vi "_API_BINANCE_GET_BookTicker.vi"(0 "BinanceAPI in":refnum<class "BinanceAPI_.lvclass">, 5 "bookTicker":cluster{"symbol (eg. BTCUSDT)":string}={"symbol (eg. BTCUSDT)"="CAKEUSDT"}, 11 "error in (no error)":errorcluster) -> (4 "BinanceAPI out":refnum<class "BinanceAPI_.lvclass">, 6 "bookTicker":T1, 14 "Body":string, 15 "error out":errorcluster)   [LabVIEW 2022 SP3, in "BinanceAPI_.lvclass"]
doc: "https://binance-docs.github.io/apidocs/spot/en/#symbol-order-book-ticker"
uses:
  BinanceAPI_.lvclass
  BinanceAPI_.lvclass/BinanceAPI_.ctl
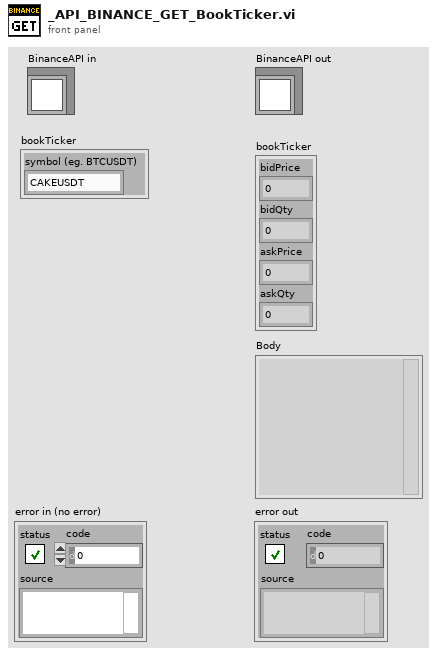
[diagram p1: front panel]
types:
  T1 = cluster{"bidPrice":dbl, "bidQty":dbl, "askPrice":dbl, "askQty":dbl}
  T2 = cluster{"bidPrice":string, "bidQty":string, "askPrice":string, "askQty":string}
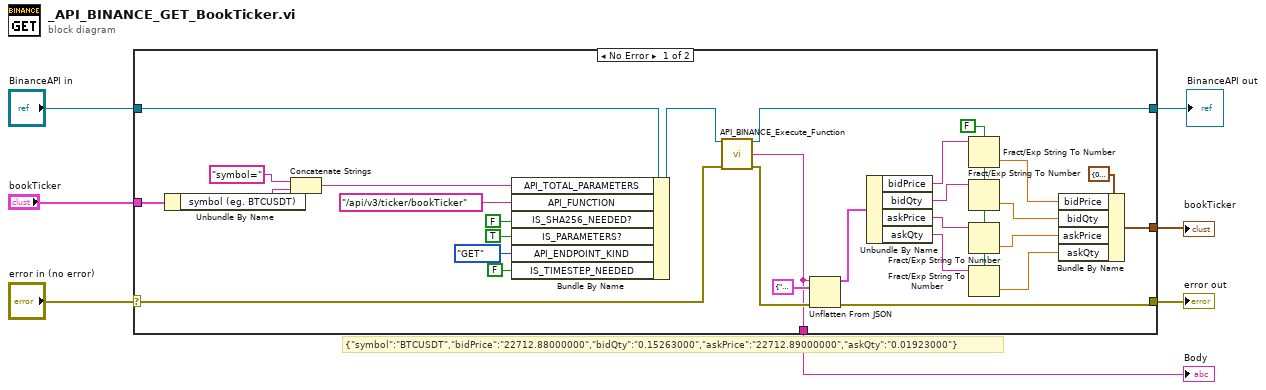
[diagram p0: block diagram]
diagram:
  # "{\"symbol\":\"BTCUSDT\",\"bidPrice\":\"22712.88000000\",\"bidQty\":\"0.15263000\",\"askPrice\":\"22712.89000000\",\"askQty\":\"0.01923000\"}"
  n1 = case shown="No Error" "error in (no error)" {
    selector: "error in (no error)" -> [w24 w38]
    tunnel: [w22 w38] -> w6
    tunnel: [w25 w37] -> w1
    tunnel: "BinanceAPI in" -> [w36 w37]
    tunnel: "bookTicker" -> [w31 _]
    tunnel: [w9 _] -> w4
    tunnel: [w8 _] -> w3
    frame No Error {
      w15 = FALSE ("use system decimal point (T)")
      n2 = Unbundle By Name(w31) -> ("symbol (eg. BTCUSDT)"=w30:string)
      n3 = Concatenate Strings("symbol=", w30) -> (w29:string)
      n4 = Bundle By Name(cluster=w36, "API_TOTAL_PARAMETERS"=w29, "API_FUNCTION"="/api/v3/ticker/bookTicker", "IS_SHA256_NEEDED?"=FALSE, "IS_PARAMETERS?"=TRUE, "API_ENDPOINT_KIND"=enum16{"POST", "DELETE", "GET", "PUT"}."GET", "IS_TIMESTEP_NEEDED"=FALSE) -> (w26:refnum<class "BinanceAPI_.lvclass">)
      n5 = call "API_BINANCE_Execute_Function.vi"("BinanceAPI in"=w26, "error in (no error)"=w24) -> ("BinanceAPI out"=w25:refnum<class "BinanceAPI_.lvclass">, "Body"=w8:string, "error out"=w23:errorcluster)  [unwired: 9 in, 2 out]
      n6 = Unflatten From JSON(JSON string=w8, type and defaults=T2 {"bidPrice"="", "bidQty"="", "askPrice"="", "askQty"=""}, error in (no error)=w23) -> (value=w20:T2, error out=w22:errorcluster)  [unwired: 4 in]
      n7 = Unbundle By Name(w20) -> ("bidPrice"=w19:string, "bidQty"=w18:string, "askPrice"=w17:string, "askQty"=w16:string)
      n8 = Fract/Exp String To Number(use system decimal point (T)=w15, string=w19) -> (number=w13:dbl)  [unwired: 2 in, 1 out]
      n9 = Fract/Exp String To Number(use system decimal point (T)=w15, string=w18) -> (number=w12:dbl)  [unwired: 2 in, 1 out]
      n10 = Fract/Exp String To Number(use system decimal point (T)=w15, string=w17) -> (number=w11:dbl)  [unwired: 2 in, 1 out]
      n11 = Fract/Exp String To Number(use system decimal point (T)=w15, string=w16) -> (number=w10:dbl)  [unwired: 2 in, 1 out]
      n12 = Bundle By Name(cluster=T1 {"bidPrice"=0.0, "bidQty"=0.0, "askPrice"=0.0, "askQty"=0.0} ("type and defaults"), "bidPrice"=w13, "bidQty"=w12, "askPrice"=w11, "askQty"=w10) -> (w9:T1)
    }
    frame Error {
    }
  }
  "error out" <- w6
  "bookTicker" <- w4
  "Body" <- w3
  "BinanceAPI out" <- w1
